vi "Configure Edge Trigger.vi"(0 "device session in":refnum<class "Device Session.lvclass">, 1 "trigger source":u8, 5 "trigger slope":T1, 7 "trigger level (V)":dbl, 9 "hysteresis (%fs)":dbl=0.25, 11 "error in":errorcluster, 12 "instance":enum16{"A", "B"}(ring)) -> (4 "device session out":refnum<class "Device Session.lvclass">, 15 "error out":errorcluster)   [LabVIEW 2021, in "Device Session.lvclass"]
doc: "Configures the edge trigger for the selected channel. You can specify the trigger level, hysteresis, and trigger slope.\n\n<B>Input Parameters</B>\n\n<B>device session in</B> is a reference to the Device Session object, which contains a session to each instrument design library used in this sample project. This parameter is obtained from the 'Open Session' VI.\n\n<B>trigger source</B> specifies the channel to monitor for trigger conditions.\n\n<B>trigger slope</B> specifies whether the oscilloscope should trigger on a rising edge or a falling edge.\n\n<B>trigger level (V)</B> specifies the voltage threshold for the trigger.\n\n<B>hysteresis (%fs)</B> specifies in volts the size of the hysteresis window on either side of the specified 'level'. The oscilloscope triggers when the 'trigger source' signal passes through the 'hysteresis level' you specify with this parameter, has the specified 'trigger slope', and passes through the specified 'level'.\n\n<B>instance</B> specifies either instance A or B of the trigger to use.\n\n<B>error in</B> describes error conditions that occur before this node runs. This input provides standard 'error in' functionality.\n\n<B>Output Parameters</B>\n\n<B>device session out</B> passes a reference to the session to the next VI.\n\n<B>error out</B> contains error information. This output provides standard 'error out' functionality."
uses:
  Device Session.lvclass
  <instrlib>/_niInstr/Data Trigger/v1/Shared/Public/Edge Configuration Trigger Slope.ctl
  Device Session.lvclass/Device Session.ctl
  <instrlib>/_niInstr/Data Trigger/v1/Shared/Public/Edge Configuration FXP(+-,18,1).ctl
  <vilib>/Utility/error.llb/Error Cluster From Error Code.vi
  <vilib>/rvi/errors/niLvFpgaAdjustHostInterfaceError.vi
  <vilib>/rvi/interface/nirviReadWriteControl/nirviReadWriteControl.xnode
  FPGA Refnum.ctl
  <vilib>/rvi/interface/Simulation/niFpgaSimulationCallBeginRW.vi
  <instrlib>/_niInstr/Data Trigger/v1/Shared/niInstr Data Trigger v1 Shared.lvlib
  NiFpgaLv.dll
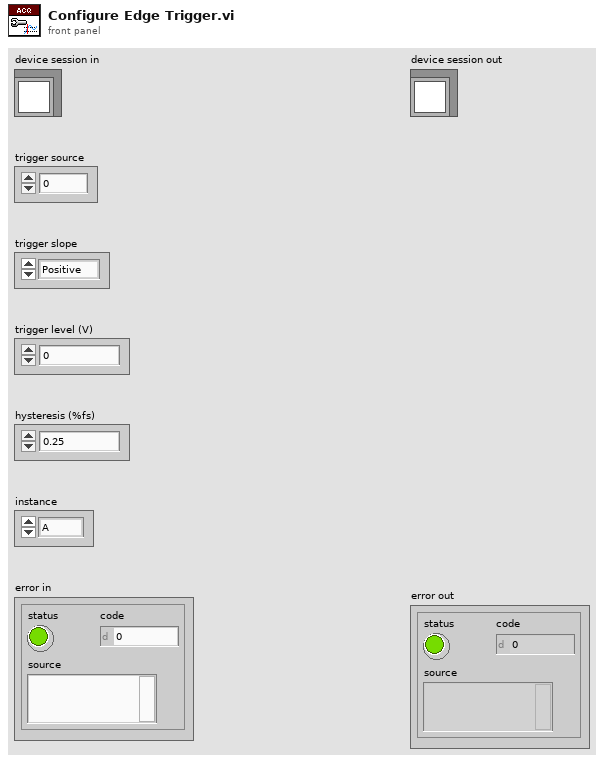
[diagram p1: front panel]
types:
  T1 = typedef "niInstr Data Trigger v1 Shared.lvlib/Edge Configuration Trigger Slope.ctl" = enum8{"Positive", "Negative"}
  T2 = typedef "niInstr Data Trigger v1 Shared.lvlib/Edge Configuration FXP(+-,18,1).ctl" = cluster{"highLevel":fxp<+/-,18,1>, "lowLevel":fxp<+/-,18,1>, "trigger slope":T1}
  T3 = enum16{"Immediate", "A", "B", "OR", "AND", "A THEN B", "B THEN A", "High Resolution"}
  T4 = typedef "Device Session.lvclass/Device Session Object.ctl" = cluster{"fpga reference":T5, "reg bus":refnum<class "niInstr FIFO Register Bus v1 Host.lvclass">, "subsystem map":refnum<class "niInstr Subsystem Map v1 Host.lvclass">, "cal data":refnum<class "niHSAI Cal Data v1 Host.lvclass">, "config":refnum<class "niHSAI Group A Config v1 Host.lvclass">, "acquisition 0":refnum<class "niInstr Multirecord Acquisition v1 Host.lvclass">, "acquisition 1":refnum<class "niInstr Multirecord Acquisition v1 Host.lvclass">, "number of selected acq channels":u8, "selected acq channels":bool[], "number of channels":u32, "configured channels":bool[], "acq configuration":cluster{"number of samples":u64, "number of records":u64, "pretrigger samples":u64}, "actual channel configuration":T6[], "sample clock rate (Hz)":dbl, "scaling coefficients":T10[]}
  T5 = typedef "Device Session.lvclass/FPGA Refnum.ctl" = refnum<k20>
  T6 = typedef "niHSAI Types v1 Host.lvlib/Channel Configuration.ctl" = cluster{"channel":u32, "coupling":T7, "impedance":T8, "bandwidth":T9, "vertical range":dbl, "vertical offset":dbl}
  T7 = typedef "niHSAI Types v1 Host.lvlib/Coupling.ctl" = enum8{"Default", "DC", "AC"}
  T8 = typedef "niHSAI Types v1 Host.lvlib/Impedance.ctl" = enum8{"Default", "1 mega ohm", "50 ohm"}
  T9 = typedef "niHSAI Types v1 Host.lvlib/Bandwidth.ctl" = enum8{"Default", "Full Bandwidth", "Anti-alias Filter", "150 MHz"}
  T10 = typedef "niInstr Multirecord Acquisition v1 Host.lvclass/Scaling Coefficient.ctl" = cluster{"gain":dbl, "offset":dbl}
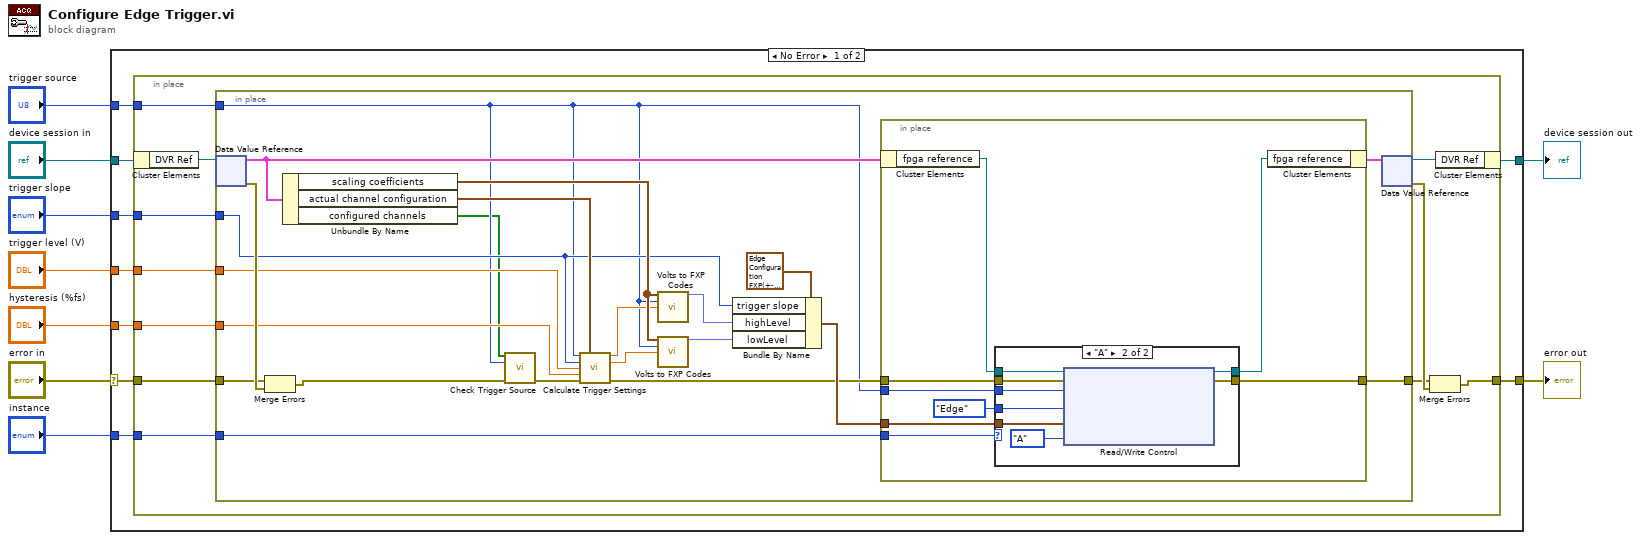
[diagram p0: block diagram]
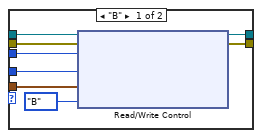
[diagram p2: hidden frame]
diagram:
  n1 = case shown="No Error" "error in" {
    selector: "error in" -> [w18 w77]
    tunnel: "device session in" -> [w11 w76]
    tunnel: [w10 w76] -> w8
    tunnel: [w12 w77] -> w9
    tunnel: "trigger source" -> [w17 _]
    tunnel: "trigger slope" -> [w16 _]
    tunnel: "trigger level (V)" -> [w15 _]
    tunnel: "hysteresis (%fs)" -> [w14 _]
    tunnel: "instance" -> [w13 _]
    frame No Error {
      n2 = in-place {
        in-place-border: w18 -> [w29]
        in-place-border: w17 -> [w28]
        in-place-border: w16 -> [w27]
        in-place-border: w15 -> [w26]
        in-place-border: w14 -> [w25]
        in-place-border: w13 -> [w23]
        in-place-border: [w21] -> w12
        n3 = in-place-cluster #1(w11) -> ("DVR Ref"=w20:refnum<data-value>)
        n4 = in-place {
          in-place-border: w29 -> [w50]
          in-place-border: w28 -> [w32]
          in-place-border: w27 -> [w34]
          in-place-border: w26 -> [w39]
          in-place-border: w25 -> [w38]
          in-place-border: w23 -> [w49]
          in-place-border: [w48] -> w22
          n5 = in-place-dvr #2(w20) -> (w36:T4, w51:errorcluster)
          n6 = Merge Errors(w50, w51) -> (w37:errorcluster)
          n7 = Unbundle By Name(w36) -> ("scaling coefficients"=w41:T10[], "actual channel configuration"=w42:T6[], "configured channels"=w30:bool[])
          n8 = call "Check Trigger Source.vi"("configured channels"=w30, "trigger source"=w32, "error in"=w37) -> ("error out"=w44:errorcluster)  [unwired: 12 in]
          n9 = call "Calculate Trigger Settings.vi"("trigger source"=w32, "actual channel configuration"=w42, "trigger slope"=w34, "level (V)"=w39, "hysteresis (%fs)"=w38, "error in"=w44) -> ("high level (V)"=w33:dbl, "low level (V)"=w40:dbl, "error out"=w43:errorcluster)  [unwired: 7 in]
          n10 = call "Volts to FXP Codes.vi"("scaling coefficients"=w41, "channel index"=w32, "level (V)"=w33) -> ("codes"=w31:fxp<+/-,18,1>)  [unwired: 12 in]
          n11 = call "Volts to FXP Codes.vi"("scaling coefficients"=w41, "channel index"=w32, "level (V)"=w40) -> ("codes"=w45:fxp<+/-,18,1>)  [unwired: 12 in]
          n12 = Bundle By Name(cluster=T2 {"highLevel"=0.0, "lowLevel"=0.0, "trigger slope"=enum."Positive"} ("configuration"), "trigger slope"=w34, "highLevel"=w31, "lowLevel"=w45) -> (w47:T2)
          n13 = in-place {
            in-place-border: w49 -> [w58]
            in-place-border: [w57] -> w48
            in-place-border: w47 -> [w56]
            in-place-border: w43 -> [w55]
            in-place-border: w32 -> [w54]
            n14 = in-place-cluster #3(w36) -> ("fpga reference"=w53:T5)
            n15 = case shown="\"A\"" w58 {
              tunnel: w55 -> [w67 w75]
              tunnel: w54 -> [w63 w71]
              tunnel: [w66 w74] -> w57
              tunnel: enum16{"Edge", "Level", "Custom"}."Edge" ("trigger.select 0") -> [w65 w73]
              tunnel: w56 -> [w64 w72]
              tunnel: w53 -> [w61 w68]
              tunnel: [w60 w69] -> w52
              frame "B" {
                n16 = xnode "Read/Write Control"("FPGA VI Reference In"=w61, "error in"=w67, "trigger.channel B"=w63, "trigger.type B"=w65, "trigger.edge B"=w64, "trigger.combination type"=T3."B" ("trigger.combination.type")) -> ("FPGA VI Reference Out"=w60:T5, "error out"=w66:errorcluster)
              }
              frame "A" {
                n17 = xnode "Read/Write Control"("FPGA VI Reference In"=w68, "error in"=w75, "trigger.channel A"=w71, "trigger.type A"=w73, "trigger.edge A"=w72, "trigger.combination type"=T3."A" ("trigger.combination.type")) -> ("FPGA VI Reference Out"=w69:T5, "error out"=w74:errorcluster)
              }
            }
            n18 = in-place-cluster #3("fpga reference"=w52) -> (w35:T4)
          }
          n19 = in-place-dvr #2(w35) -> (w19:refnum<data-value>, w24:errorcluster)
        }
        n20 = Merge Errors(w22, w24) -> (w21:errorcluster)
        n21 = in-place-cluster #1("DVR Ref"=w19) -> (w10:refnum<class "Device Session.lvclass">)
      }
    }
    frame Error {
    }
  }
  "error out" <- w9
  "device session out" <- w8
